vi "SQLite_Return_Code.vi"(8 "Return_Code":i32, 9 "error in (no error)":errorcluster) -> (0 "error out":errorcluster)   [LabVIEW 2020, in "SQLiteBase.lvlib"]
uses:
  SQLiteBase.lvlib
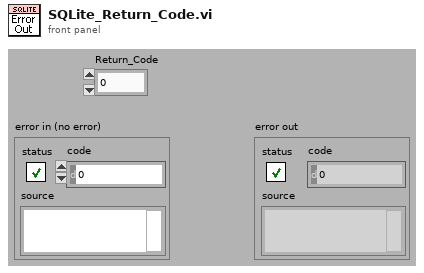
[diagram p1: front panel]
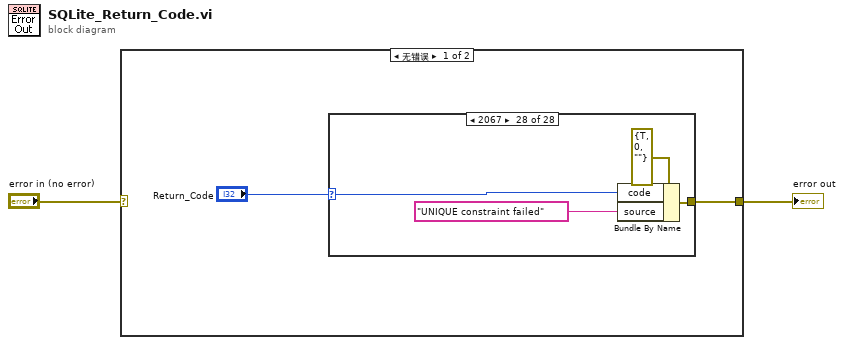
[diagram p0: block diagram]
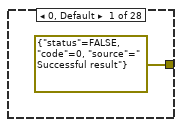
[diagram p2: hidden frame]
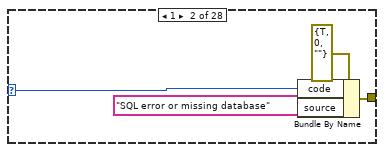
[diagram p3: hidden frame]
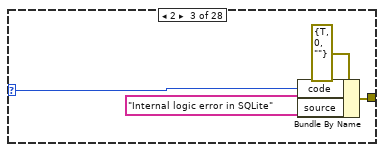
[diagram p4: hidden frame]
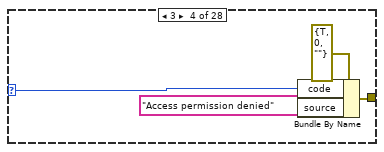
[diagram p5: hidden frame]
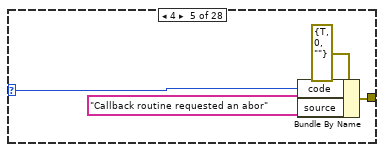
[diagram p6: hidden frame]
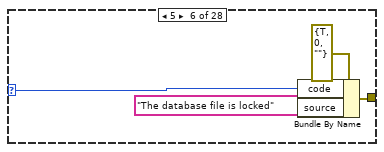
[diagram p7: hidden frame]
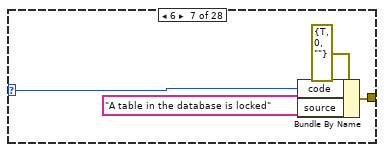
[diagram p8: hidden frame]
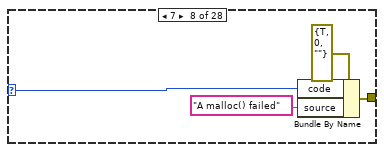
[diagram p9: hidden frame]
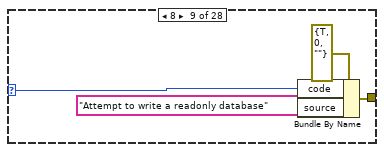
[diagram p10: hidden frame]
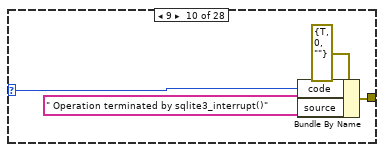
[diagram p11: hidden frame]
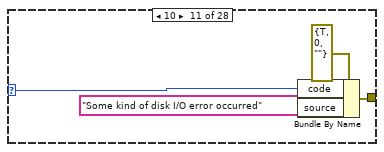
[diagram p12: hidden frame]
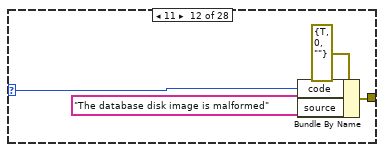
[diagram p13: hidden frame]
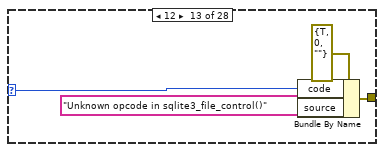
[diagram p14: hidden frame]
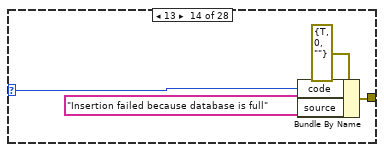
[diagram p15: hidden frame]
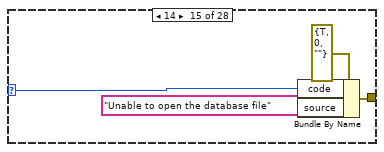
[diagram p16: hidden frame]
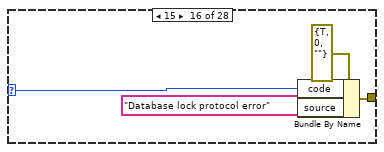
[diagram p17: hidden frame]
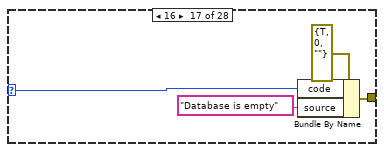
[diagram p18: hidden frame]
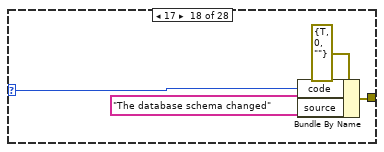
[diagram p19: hidden frame]
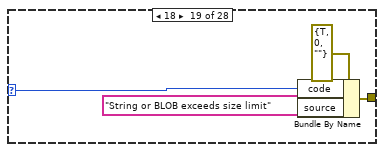
[diagram p20: hidden frame]
diagram:
  n1 = case shown="无错误" "error in (no error)" {
    selector: "error in (no error)" -> [_ w114]
    tunnel: [w4 w114] -> w2
    frame No Error {
      n2 = case shown="2067" "Return_Code" {
        selector: "Return_Code" -> [_ w7 w11 w15 w19 w23 w27 w31 w35 w39 w43 w47 w51 w55 w59 w63 w67 w71 w75 w79 w83 w87 w91 w95 w99 w103 w107 w111]
        tunnel: [errorcluster {"status"=FALSE, "code"=0, "source"=" Successful result"} ("error out") w8 w12 w16 w20 w24 w28 w32 w36 w40 w44 w48 w52 w56 w60 w64 w68 w72 w76 w80 w84 w88 w92 w96 w100 w104 w108 w112] -> w4
        frame 0, Default {
        }
        frame 1 {
          n3 = Bundle By Name(cluster=errorcluster {"status"=TRUE, "code"=0, "source"=""} ("error out"), "code"=w7, "source"="SQL error or missing database") -> (w8:errorcluster)
        }
        frame 2 {
          n4 = Bundle By Name(cluster=errorcluster {"status"=TRUE, "code"=0, "source"=""} ("error out"), "code"=w11, "source"="Internal logic error in SQLite") -> (w12:errorcluster)
        }
        frame 3 {
          n5 = Bundle By Name(cluster=errorcluster {"status"=TRUE, "code"=0, "source"=""} ("error out"), "code"=w15, "source"="Access permission denied") -> (w16:errorcluster)
        }
        frame 4 {
          n6 = Bundle By Name(cluster=errorcluster {"status"=TRUE, "code"=0, "source"=""} ("error out"), "code"=w19, "source"="Callback routine requested an abor") -> (w20:errorcluster)
        }
        frame 5 {
          n7 = Bundle By Name(cluster=errorcluster {"status"=TRUE, "code"=0, "source"=""} ("error out"), "code"=w23, "source"="The database file is locked") -> (w24:errorcluster)
        }
        frame 6 {
          n8 = Bundle By Name(cluster=errorcluster {"status"=TRUE, "code"=0, "source"=""} ("error out"), "code"=w27, "source"="A table in the database is locked") -> (w28:errorcluster)
        }
        frame 7 {
          n9 = Bundle By Name(cluster=errorcluster {"status"=TRUE, "code"=0, "source"=""} ("error out"), "code"=w31, "source"="A malloc() failed") -> (w32:errorcluster)
        }
        frame 8 {
          n10 = Bundle By Name(cluster=errorcluster {"status"=TRUE, "code"=0, "source"=""} ("error out"), "code"=w35, "source"="Attempt to write a readonly database") -> (w36:errorcluster)
        }
        frame 9 {
          n11 = Bundle By Name(cluster=errorcluster {"status"=TRUE, "code"=0, "source"=""} ("error out"), "code"=w39, "source"=" Operation terminated by sqlite3_interrupt()") -> (w40:errorcluster)
        }
        frame 10 {
          n12 = Bundle By Name(cluster=errorcluster {"status"=TRUE, "code"=0, "source"=""} ("error out"), "code"=w43, "source"="Some kind of disk I/O error occurred") -> (w44:errorcluster)
        }
        frame 11 {
          n13 = Bundle By Name(cluster=errorcluster {"status"=TRUE, "code"=0, "source"=""} ("error out"), "code"=w47, "source"="The database disk image is malformed") -> (w48:errorcluster)
        }
        frame 12 {
          n14 = Bundle By Name(cluster=errorcluster {"status"=TRUE, "code"=0, "source"=""} ("error out"), "code"=w51, "source"="Unknown opcode in sqlite3_file_control()") -> (w52:errorcluster)
        }
        frame 13 {
          n15 = Bundle By Name(cluster=errorcluster {"status"=TRUE, "code"=0, "source"=""} ("error out"), "code"=w55, "source"="Insertion failed because database is full") -> (w56:errorcluster)
        }
        frame 14 {
          n16 = Bundle By Name(cluster=errorcluster {"status"=TRUE, "code"=0, "source"=""} ("error out"), "code"=w59, "source"="Unable to open the database file") -> (w60:errorcluster)
        }
        frame 15 {
          n17 = Bundle By Name(cluster=errorcluster {"status"=TRUE, "code"=0, "source"=""} ("error out"), "code"=w63, "source"="Database lock protocol error") -> (w64:errorcluster)
        }
        frame 16 {
          n18 = Bundle By Name(cluster=errorcluster {"status"=TRUE, "code"=0, "source"=""} ("error out"), "code"=w67, "source"="Database is empty") -> (w68:errorcluster)
        }
        frame 17 {
          n19 = Bundle By Name(cluster=errorcluster {"status"=TRUE, "code"=0, "source"=""} ("error out"), "code"=w71, "source"="The database schema changed") -> (w72:errorcluster)
        }
        frame 18 {
          n20 = Bundle By Name(cluster=errorcluster {"status"=TRUE, "code"=0, "source"=""} ("error out"), "code"=w75, "source"="String or BLOB exceeds size limit") -> (w76:errorcluster)
        }
        frame 19 {
          n21 = Bundle By Name(cluster=errorcluster {"status"=TRUE, "code"=0, "source"=""} ("error out"), "code"=w79, "source"="Abort due to constraint violation") -> (w80:errorcluster)
        }
        frame 20 {
          n22 = Bundle By Name(cluster=errorcluster {"status"=TRUE, "code"=0, "source"=""} ("error out"), "code"=w83, "source"="Data type mismatch") -> (w84:errorcluster)
        }
        frame 21 {
          n23 = Bundle By Name(cluster=errorcluster {"status"=TRUE, "code"=0, "source"=""} ("error out"), "code"=w87, "source"="Library used incorrectly") -> (w88:errorcluster)
        }
        frame 22 {
          n24 = Bundle By Name(cluster=errorcluster {"status"=TRUE, "code"=0, "source"=""} ("error out"), "code"=w91, "source"="Uses OS features not supported on host") -> (w92:errorcluster)
        }
        frame 23 {
          n25 = Bundle By Name(cluster=errorcluster {"status"=TRUE, "code"=0, "source"=""} ("error out"), "code"=w95, "source"=" Authorization denied") -> (w96:errorcluster)
        }
        frame 24 {
          n26 = Bundle By Name(cluster=errorcluster {"status"=TRUE, "code"=0, "source"=""} ("error out"), "code"=w99, "source"="Auxiliary database format error") -> (w100:errorcluster)
        }
        frame 25 {
          n27 = Bundle By Name(cluster=errorcluster {"status"=TRUE, "code"=0, "source"=""} ("error out"), "code"=w103, "source"="2nd parameter to sqlite3_bind out of range") -> (w104:errorcluster)
        }
        frame 26 {
          n28 = Bundle By Name(cluster=errorcluster {"status"=TRUE, "code"=0, "source"=""} ("error out"), "code"=w107, "source"=" File opened that is not a database file ") -> (w108:errorcluster)
        }
        frame 2067 {
          n29 = Bundle By Name(cluster=errorcluster {"status"=TRUE, "code"=0, "source"=""} ("error out"), "code"=w111, "source"="UNIQUE constraint failed") -> (w112:errorcluster)
        }
      }
    }
    frame Error {
    }
  }
  "error out" <- w2
